vi "Write Result.vi"(0 "Vector Charact Result Accessor in":refnum<class "Vector Charact Result Accessor.lvclass">, 5 "Charact Result":variant, 11 "error in":errorcluster) -> (4 "Vector Charact Result Accessor out":refnum<class "Vector Charact Result Accessor.lvclass">, 15 "error out":errorcluster)   [LabVIEW 2023, in "RFFixtureCharact.Public.lvlib" / "Vector Charact Result Accessor.lvclass"]
uses:
  Vector Charact Result Accessor.lvclass
  C:/rfcal/AuxTools/STSRFFixtureCharactUtility/Source/Code Modules/Fixture/RMM/Charact Result Accessor/Base/Charact Result Accessor.lvclass
  <vilib>/addons/_RFCalAndCharactDatabase/NI_RFCalAndCharact_Database_API.lvlibp/Characterization/Controls/Type.ctl
  Base Classes/Vector/Vector Abstract Path/Type Definitions/Vector Charact Result.ctl
  Vector Charact Result Accessor.lvclass/Vector Charact Result Accessor.ctl
  <vilib>/addons/_RFCalAndCharactDatabase/NI_RFCalAndCharact_Database_API.lvlibp/Characterization/Characterization.lvlib
  Base Classes/Vector/Vector Abstract Path/Vector Abstract Path.lvclass
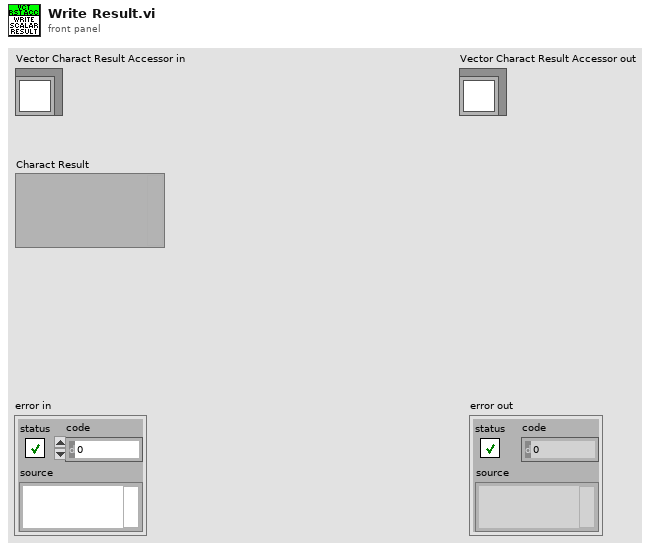
[diagram p1: front panel]
types:
  T1 = typedef "RFFixtureCharact.Public.lvlib/Vector Abstract Path.lvclass/Vector Charact Result.ctl" = cluster{"Port Power":dbl, "Frequency":dbl, "S Parameters":cdb[], "Out Of Limit":bool}
  T2 = typedef "NI_RFCalAndCharact_Database_API.lvlibp/Characterization.lvlib/Type.ctl" = u16
  T3 = typedef "NI_RFCalAndCharact_Database_API.lvlibp/Characterization.lvlib/Path Handle.ctl" = refnum<k24>
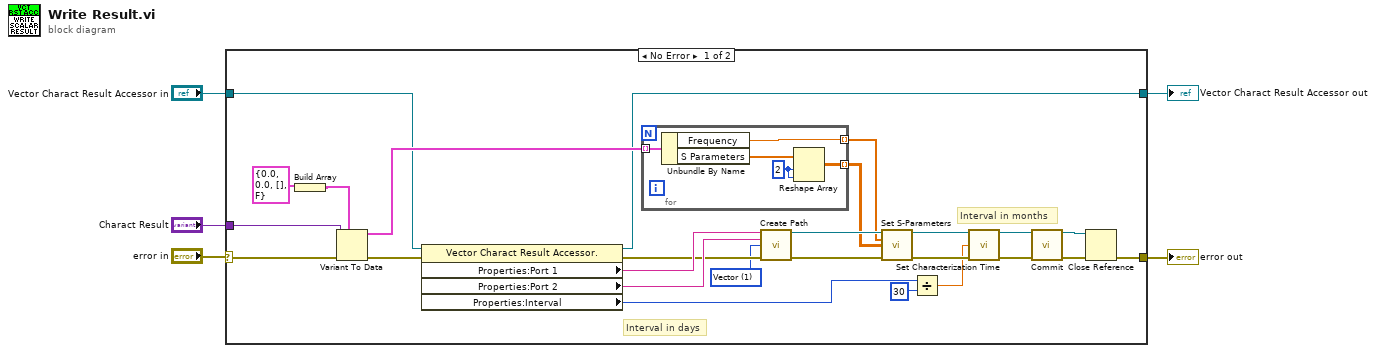
[diagram p0: block diagram]
diagram:
  n1 = case shown="No Error" "error in" {
    selector: "error in" -> [w31 w38]
    tunnel: [w12 w38] -> w1
    tunnel: "Charact Result" -> [w30 _]
    tunnel: "Vector Charact Result Accessor in" -> [w27 w37]
    tunnel: [w11 w37] -> w2
    frame No Error {
      w23 = T2 1 items=["Scalar", "Vector"] ("Type")
      # "Interval in months"
      # "Interval in days"
      n2 = Build Array(T1 {"Port Power"=0.0, "Frequency"=0.0, "S Parameters"=[], "Out Of Limit"=FALSE} ("Cal Result")) -> (w6:T1[])
      n3 = Variant To Data(error in=w31, type=w6, Variant=w30) -> (data=w29:T1[], error out=w28:errorcluster)
      n4 = property class="Vector Charact Result Accessor."(reference=w27, error in=w28) -> (reference out=w11:refnum<class "Vector Charact Result Accessor.lvclass">, error out=w24:errorcluster, "Properties:Port 1"=w26:string, "Properties:Port 2"=w25:string, "Properties:Interval"=w10:i32)
      n5 = for {
        tunnel: w29 -> [w36] mode=indexing
        tunnel: [w35] -> w18 mode=indexing
        tunnel: [w32] -> w17 mode=indexing
        w33 = 2 ("dimension size")
        n6 = Unbundle By Name(w36) -> ("Frequency"=w35:dbl, "S Parameters"=w34:cdb[])
        n7 = Reshape Array(w34, w33, w33) -> (w32:cdb[][])
      }
      n8 = call <vilib>:"Create Path.vi"("Port 1"=w26, "Port 2"=w25, "Type"=w23, "error in"=w24) -> ("Path"=w19:T3, "error out"=w22:errorcluster)  [unwired: 10 in]
      n9 = call <vilib>:"Set S-Parameters.vi"("Path In"=w19, "Frequencies (Hz)"=w18, "S-Parameters"=w17, "error in"=w22) -> ("Path Out"=w20:T3, "error out"=w21:errorcluster)  [unwired: 10 in]
      n10 = Divide(x=w10, y=30) -> (x/y=w8:dbl)
      n11 = call <vilib>:"Set Characterization Time.vi"("Path In"=w20, "Interval (Months)"=w8, "error in"=w21) -> ("Path Out"=w15:T3, "error out"=w16:errorcluster)  [unwired: 11 in]
      n12 = call <vilib>:"Commit.vi"("Path In"=w15, "error in"=w16) -> ("Path Out"=w13:T3, "error out"=w14:errorcluster)  [unwired: 12 in]
      n13 = Close Reference(reference=w13, error in (no error)=w14) -> (error out=w12:errorcluster)
    }
    frame Error {
    }
  }
  "error out" <- w1
  "Vector Charact Result Accessor out" <- w2
